vi "API - Transient - Capture Transients.vi"(8 "error in":errorcluster, 9 "Soft Trigger":bool=TRUE, 10 "Maximum Waveform Length":i32=10000, 11 "configuration file path":path) -> (0 "error out":errorcluster)   [LabVIEW 2017, in "DTACQ - Network Enabled Device Driver.lvlib"]
doc: "Captures transient data and publishes that data to a shared variable"
uses:
  DTACQ - Network Enabled Device Driver.lvlib
  Close Transient Mode.vi
  Read Transient Data and Write to Shared Variable.vi
  Fire Transient.vi
  Arm and Set Trigger - Transient.vi
  Initialise Transient Mode.vi
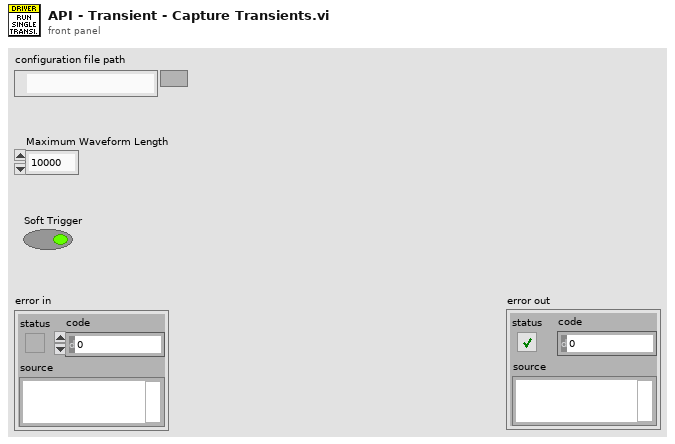
[diagram p1: front panel]
types:
  T1 = typedef "Communications Library.lvlib/DTACQ Connection Data--Cluster.ctl" = cluster{"Description":string, "Address":string, "Port":u16, "timeout (ms)":i32, "Termination Character":string, "TCP Connection Reference":refnum<k5>, "Open Connection":bool}
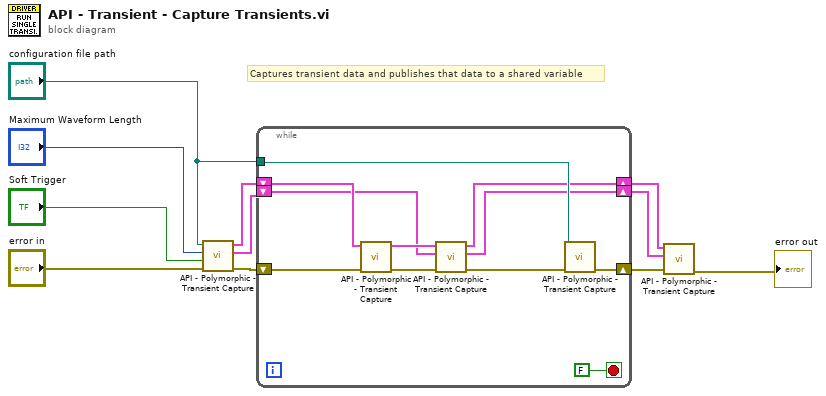
[diagram p0: block diagram]
diagram:
  # "Captures transient data and publishes that data to a shared variable"
  n1 = call-poly "API - Polymorphic - Transient Capture.vi"("error in"="error in", "Soft Trigger"="Soft Trigger", "Maximum Waveform Length"="Maximum Waveform Length", "configuration file path"="configuration file path") -> ("error out"=w11:errorcluster, "AI Connection Out"=w5:T1, "Carrier Connection Out"=w7:T1)  [unwired: 5 in]
  n2 = while {
    tunnel: "configuration file path" -> [w17]
    shift-right: [w22] -> w4
    shift-left: w11 -> [w21]
    shift-right: [w13] -> w3
    shift-left: w7 -> [w20]
    shift-right: [w12] -> w2
    shift-left: w5 -> [w15]
    stop <- FALSE stop-if-true
    n3 = call-poly "API - Polymorphic - Transient Capture.vi"("error in"=w21, "Carrier Connection In"=w20) -> ("error out"=w19:errorcluster, "DTACQ Connection Out"=w18:T1)  [unwired: 8 in]
    n4 = call-poly "API - Polymorphic - Transient Capture.vi"("error in"=w19, "AI Connection In"=w15, "Carrier Connection In"=w18) -> ("error out"=w16:errorcluster, "AI Connection Out"=w12:T1, "Carrier Connection Out"=w13:T1)  [unwired: 6 in]
    n5 = call-poly "API - Polymorphic - Transient Capture.vi"("error in"=w16, "configuration file path"=w17) -> ("error out"=w22:errorcluster)  [unwired: 9 in]
  }
  n6 = call-poly "API - Polymorphic - Transient Capture.vi"("error in"=w4, "AI TCP Connection In"=w2, "Carrier TCP Connection In"=w3) -> ("error out"=→"error out":errorcluster)  [unwired: 8 in]
